vi "ARMA Model Estimation.vi"() -> ()   [LabVIEW 2023]
doc: "This example shows how to obtain ARMA model parameters of a univariate time series using TSA ARMA Modeling VI.\n\n<b>Instructions:</b>\n1) Run this VI.\n2) Set the coefficients for the IIR filter.\n3) Observe the detected coefficients from ARMA modeling."
uses:
  <vilib>/Analysis/3filter.llb/IIR Filter (DBL).vi
  <vilib>/addons/Time Series Analysis/Modeling and Prediction.llb/TSA ARMA Modeling (Array).vi
  <vilib>/addons/_Advanced Signal Processing/NI_AdvSigProcTSA.lvlib
  <vilib>/Analysis/NI_AALBase.lvlib
panel:
  out "Time Series from the Simulated System":dbl[](graph)
  in  "stop":bool
  out "Estimated MA coefficients":dbl[](array[numeric])
  out "MA Coefficients":dbl[][](graph)
  in  "ARMA order":cluster{"AR":i32, "MA":i32}={"AR"=3, "MA"=2}
  in  "Method":u16(ring) items=["Yule-Walker", "High order AR", "Polynomial"]
  in  "Reverse coefficients":dbl[](array[numeric])=[1.0, -1.52, 1.112, -0.4]
  in  "Forward coefficients":dbl[](array[numeric])=[1.0, 0.35, -0.5]
  out "Estimated AR coefficients":dbl[](array[numeric])
  out "AR Coefficients":dbl[][](graph)
  # "Overview: Shows how to obtain ARMA model parameters of a univariate time series using TSA ARMA Modeling VI.\nRequirements: LabVIEW Full Development System, Advanced Signal Processing Toolkit\nInstructions: \n1. Run this VI.\n2. Set the coefficients for the IIR filter.\n3. Observe the detected coefficients from ARMA modeling. \n4. Click Stop to stop the VI."
  # "Simulated System (IIR Filter)"
  # "Modeling Settings"
  # "The first element of the  Reverse coefficients must be 1."
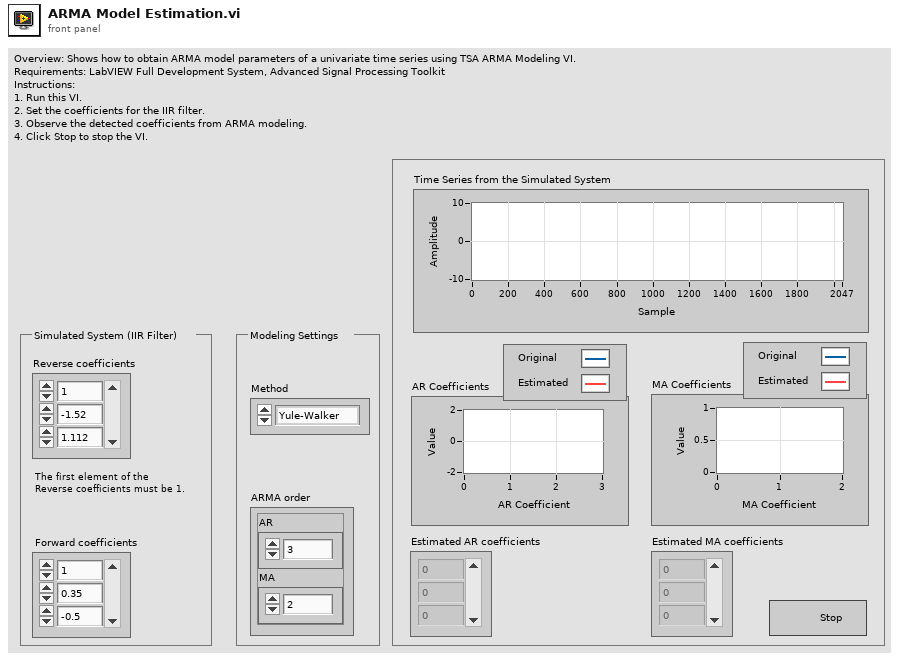
[diagram p1: front panel]
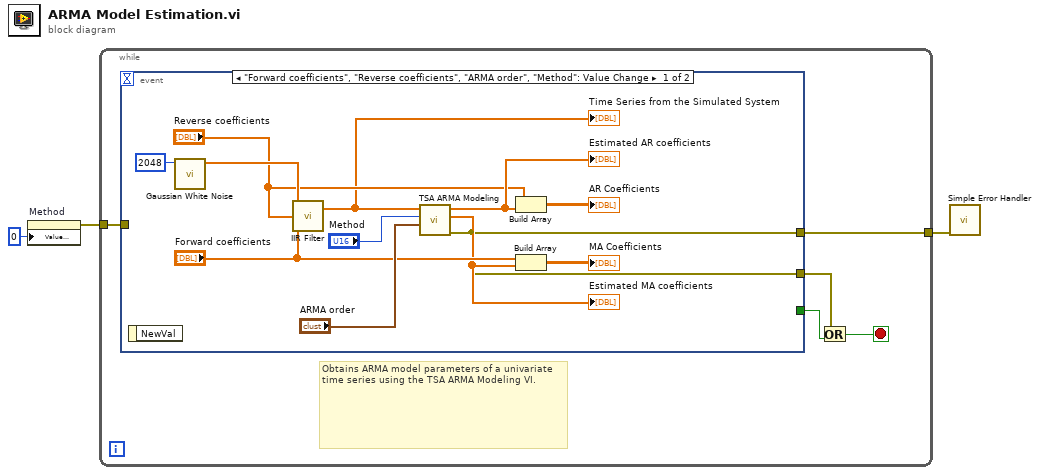
[diagram p0: block diagram]
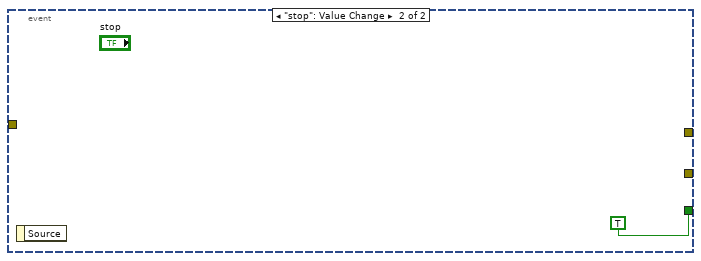
[diagram p2: hidden frame]
diagram:
  n1 = property on="Method" class="Ring (strict)"("Value (Signaling)"=u16 0) -> (error out=w2:errorcluster)  [unwired: 2 in, 1 out]
  n2 = while {
    tunnel: w2 -> [w8]
    tunnel: [w7] -> w1
    stop <- w4 stop-if-true
    # "Obtains ARMA model parameters of a univariate time series using the TSA ARMA Modeling VI."
    n3 = event shown="[0] \"Forward coefficients\", \"Reverse coefficients\", \"ARMA order\", \"Method\": Value Change" {
      selector: _ -> [_ _]
      dyn-events: _ -> [_ _]
      timeout: _ -> [_ _]
      tunnel: [_ TRUE] -> w5
      tunnel: [w9 _] -> w7
      tunnel: w8 -> [_ _]
      tunnel: [w9 _] -> w6
      event "Forward coefficients", "Reverse coefficients", "ARMA order", "Method": Value Change {
        n4 = event-data() -> ()  [unwired: 2 out]
        n5 = call <vilib>:"Gaussian White Noise.vi"("samples"=2048) -> ("Gaussian noise pattern"=w17:dbl[])  [unwired: 9 in, 1 out]
        n6 = call-poly <vilib>:"IIR Filter.vi"("Forward Coefficients"="Forward coefficients", "Reverse Coefficients"="Reverse coefficients", "X"=w17) -> ("Filtered X"=w10:dbl[])  [unwired: 1 in, 1 out]
        "Time Series from the Simulated System" <- w10
        n7 = call-poly <vilib>:"TSA ARMA Modeling.vi"("ARMA order"="ARMA order", "method"="Method", "Xt"=w10) -> ("error out"=w9:errorcluster, "MA coefficients"=w11:dbl[], "AR coefficients"=w19:dbl[])  [unwired: 1 in, 5 out]
        "Estimated AR coefficients" <- w19
        "Estimated MA coefficients" <- w11
        n8 = Build Array("Reverse coefficients", w19) -> (→"AR Coefficients":dbl[][])
        n9 = Build Array("Forward coefficients", w11) -> (→"MA Coefficients":dbl[][])
      }
      event "stop": Value Change {
        n10 = event-data() -> ()  [unwired: 2 out]
      }
    }
    n11 = Or(x=w6, y=w5) -> (x .or. y?=w4:bool)
  }
  n12 = call <vilib>:"Simple Error Handler.vi"("error in (no error)"=w1) -> ()  [unwired: 1 in, 8 out]
